vi "MW_Display_Py_Get_Frame.vi"(0 "session in":refnum<k35>, 5 "module path":path=path "D:/dev/Guy_Storage/Work/Cancun/MW_Display_Test/Magewell Capture/Capture_LV.py", 11 "error in":errorcluster, 12 "Frame Dims":T1) -> (4 "session out":refnum<k35>, 6 "module path out":path, 13 "1D Pixels":u8[](array[numeric]), 14 "RGB Pixels":u32[][](array[numeric]), 15 "error out":errorcluster)   [LabVIEW 2023]
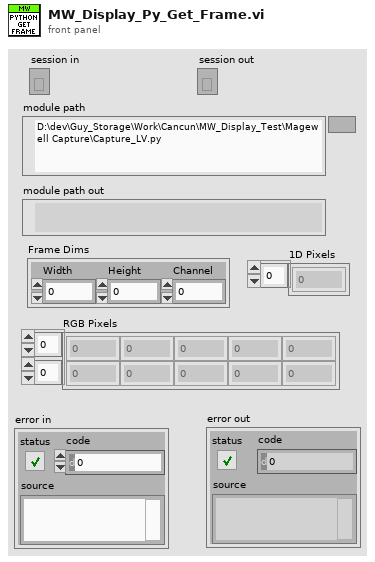
[diagram p1: front panel]
types:
  T1 = cluster{"Width":i32, "Height":i32, "Channel":i32}
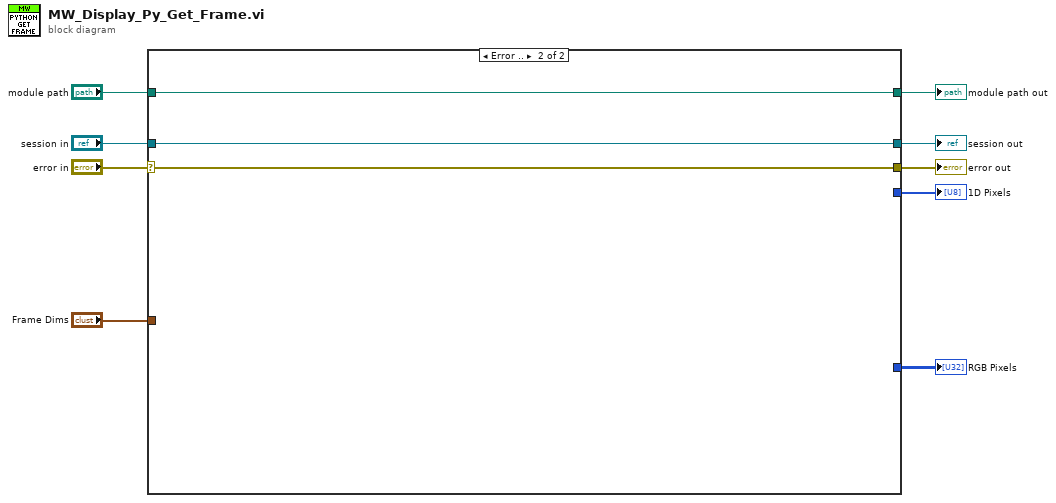
[diagram p0: block diagram]
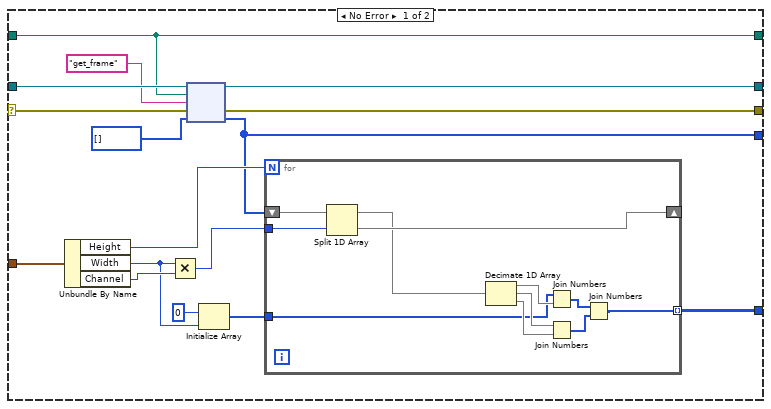
[diagram p2: hidden frame]
diagram:
  n1 = case shown="Error .." "error in" {
    selector: "error in" -> [w22 w38]
    tunnel: "module path" -> [w20 w37]
    tunnel: "session in" -> [w25 w39]
    tunnel: [w24 w38] -> w5
    tunnel: [w23 w39] -> w7
    tunnel: [w20 w37] -> w4
    tunnel: "Frame Dims" -> [w18 _]
    tunnel: [w11 _] -> w2
    tunnel: [w10 _] -> w1
    frame No Error {
      n2 = Unbundle By Name(w18) -> ("Height"=w15:i32, "Width"=w13:i32, "Channel"=w17:i32)
      n3 = Multiply(x=w13, y=w17) -> (x*y=w16:i32)
      n4 = node(w25, w20, "get_frame" ("function name"), w22, u8[] []) -> (w23:refnum<k35>, w24:errorcluster, w10:u8[])  [unwired: 2 out]
      n5 = Initialize Array(u8 0, w13) -> (w12:u8[])
      n6 = for {
        N: w15 -> [_]
        tunnel: w16 -> [w35]
        shift-right: [w34] -> _
        shift-left: w10 -> [w36]
        tunnel: [w30] -> w11 mode=indexing
        tunnel: w12 -> [w26]
        n7 = Split 1D Array(array=w36, index=w35) -> (first subarray=w33:u8[], second subarray=w34:u8[])
        n8 = Decimate 1D Array(w33) -> (w27:u8[], w29:u8[], w28:u8[])
        n9 = Join Numbers(hi=w26, lo=w27) -> ((hi.lo)=w31:u16[])
        n10 = Join Numbers(hi=w29, lo=w28) -> ((hi.lo)=w32:u16[])
        n11 = Join Numbers(hi=w31, lo=w32) -> ((hi.lo)=w30:u32[])
      }
    }
    frame Error {
    }
  }
  "session out" <- w7
  "error out" <- w5
  "module path out" <- w4
  "RGB Pixels" <- w2
  "1D Pixels" <- w1
